vi "Load and Apply Panel Layout to VI.vi"(4 "defer panel updates (F)":bool, 5 "panel layout folder (\"\")":path, 6 "bounds (panel bounds)":T1, 7 "scaling settings":T2, 8 "error in":errorcluster, 9 "keyword to match (\"\")":string, 10 "desired panel size ([-1,-1])":T4={"Horizontal"=-1, "Vertical"=-1}, 11 "VI refnum":refnum<vi>) -> (0 "error out":errorcluster, 1 "found?":bool)   [LabVIEW 2012, in "NI_SE_Front Panel Layout.lvlib"]
doc: "Find, load, and apply the best panel layout file for the VI. The panel layout file must use the naming convention:\n<b><VI name>_w<width>_h<height>_k_<keyword>.xml</b>\n<VI name>: Name of the file in <b>VI path</b> without the file extension.\n<width> and <height>: Size of the front panel used to match the optional values in <b>desired panel size</b>. If <b>desired panel size</b> is wired, then the panel layout file with the closest size values will be found. If unwired, then the panel layout file closest to the primary monitor's resolution will be found.\n<keyword>: Optional keyword used to differentiate between panel layout files. If <b>keyword to match</b> is wired, then only files with the same keyword will be found.\n\nIf <b>panel layout folder</b> is wired, this VI searches for the panel layout file in the specified folder. Otherwise, this VI searches in the folder that contains <b>VI path</b>.\n\n<b>bounds</b> determines whether the panel size or the window size is used to to set the size of the VI."
uses:
  NI_SE_Front Panel Layout.lvlib
  <vilib>/Utility/miscctls.llb/LVPointTypeDef.ctl
  Scaling Settings.ctl
  Scaling Type.ctl
  Bounds Type.ctl
  VI Panel Layout/VI Panel Layout.lvclass
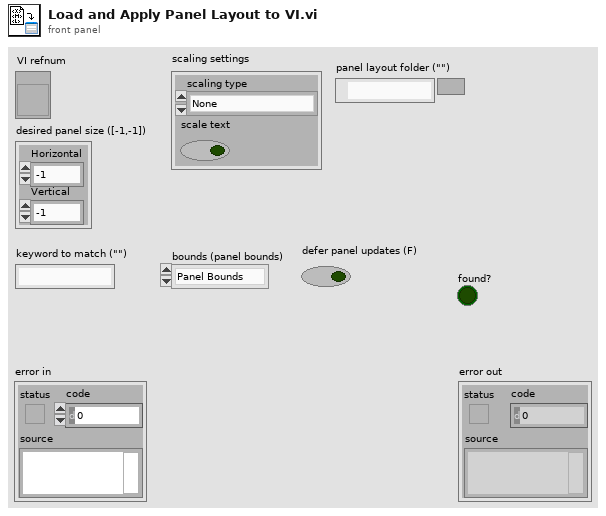
[diagram p1: front panel]
types:
  T1 = typedef "NI_SE_Front Panel Layout.lvlib/Bounds Type.ctl" = enum16{"Panel Bounds", "Window Bounds"}
  T2 = typedef "NI_SE_Front Panel Layout.lvlib/Scaling Settings.ctl" = cluster{"scaling type":T3, "scale text":bool}
  T3 = typedef "NI_SE_Front Panel Layout.lvlib/Scaling Type.ctl" = enum16{"None", "Scale panel to fit layout", "Scale layout to fit panel"}
  T4 = typedef "LVPointTypeDef.ctl" = cluster{"Horizontal":i16, "Vertical":i16}
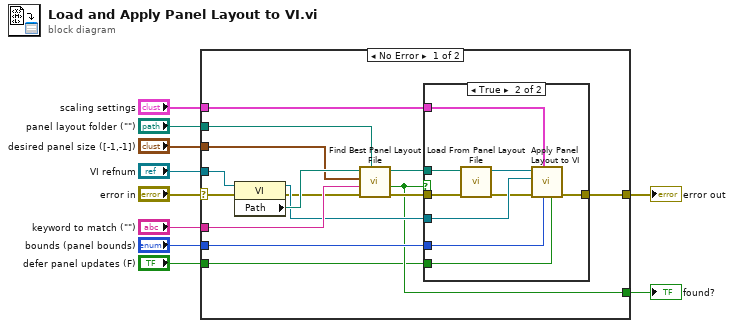
[diagram p0: block diagram]
diagram:
  n1 = case shown="No Error" "error in" {
    selector: "error in" -> [w24 w36]
    tunnel: [w12 w36] -> w9
    tunnel: "VI refnum" -> [w25 _]
    tunnel: "keyword to match (\"\")" -> [w19 _]
    tunnel: "desired panel size ([-1,-1])" -> [w20 _]
    tunnel: "scaling settings" -> [w15 _]
    tunnel: [w14 _] -> w5
    tunnel: "panel layout folder (\"\")" -> [w18 _]
    tunnel: "bounds (panel bounds)" -> [w16 _]
    tunnel: "defer panel updates (F)" -> [w11 _]
    frame No Error {
      n2 = property class="VI"(reference=w25, error in=w24) -> (reference out=w17:refnum<vi>, error out=w13:errorcluster, "Path"=w21:path)
      n3 = call "Find Best Panel Layout File.vi"("panel layout folder (\"\")"=w18, "error in"=w13, "keyword to match (\"\")"=w19, "desired panel size ([-1,-1])"=w20, "VI path"=w21) -> ("error out"=w22:errorcluster, "found?"=w14:bool, "panel layout file"=w23:path)  [unwired: 4 in]
      n4 = case shown="True" w14 {
        tunnel: w22 -> [w26 w29]
        tunnel: w23 -> [_ w31]
        tunnel: w17 -> [_ w35]
        tunnel: [w26 w34] -> w12
        tunnel: w15 -> [_ w33]
        tunnel: w16 -> [_ w28]
        tunnel: w11 -> [_ w27]
        frame False {
        }
        frame True {
          n5 = call "Load From Panel Layout File.vi"("error in"=w29, "panel layout file"=w31) -> ("error out"=w30:errorcluster, "panel layout out"=w32:refnum<class "VI Panel Layout.lvclass">)  [unwired: 8 in]
          n6 = call "Apply Panel Layout to VI.vi"("defer panel updates (F)"=w27, "bounds (panel bounds)"=w28, "scaling settings"=w33, "error in"=w30, "VI refnum"=w35, "panel layout in"=w32) -> ("error out"=w34:errorcluster)  [unwired: 4 in, 1 out]
        }
      }
    }
    frame Error {
    }
  }
  "error out" <- w9
  "found?" <- w5
